vi "LinearRegression.vi"(8 "error in":errorcluster) -> (0 "error out":errorcluster, 3 "out":refnum<class "LinearRegression.lvclass">)   [LabVIEW 2020]
doc: "Ordinary least squares Linear Regression.\n\n LinearRegression fits a linear model with coefficients w = (w1, ..., wp)\n to minimize the residual sum of squares between the observed targets in\n the dataset, and the targets predicted by the linear approximation.\n\n Parameters\n ----------\n fit_intercept : bool, default=True\n Whether to calculate the intercept for this model. If set\n to False, no intercept will be used in calculations\n (i.e. data is expected to be centered).\n\n normalize : bool, default=False\n This parameter is ignored when ``fit_intercept`` is set to False.\n If True, the regressors X will be normalized before regression by\n subtracting the mean and dividing by the l2-norm.\n If you wish to standardize, please use\n :class:`~sklearn.preprocessing.StandardScaler` before calling ``fit``\n on an estimator with ``normalize=False``.\n\n copy_X : bool, default=True\n If True, X will be copied; else, it may be overwritten.\n\n n_jobs : int, default=None\n The number of jobs to use for the computation. This will only provide\n speedup for n_targets > 1 and sufficient large problems.\n ``None`` means 1 unless in a :obj:`joblib.parallel_backend` context.\n ``-1`` means using all processors. See :term:`Glossary <n_jobs>`\n for more details.\n\n positive : bool, default=False\n When set to ``True``, forces the coefficients to be positive. This\n option is only supported for dense arrays.\n\n .. versionadded:: 0.24\n\n Attributes\n ----------\n coef_ : array of shape (n_features, ) or (n_targets, n_features)\n Estimated coefficients for the linear regression problem.\n If multiple targets are passed during the fit (y 2D), this\n is a 2D array of shape (n_targets, n_features), while if only\n one target is passed, this is a 1D array of length n_features.\n\n rank_ : int\n Rank of matrix `X`. Only available when `X` is dense.\n\n singular_ : array of shape (min(X, y),)\n Singular values of `X`. Only available when `X` is dense.\n\n intercept_ : float or array of shape (n_targets,)\n Independent term in the linear model. Set to 0.0 if\n `fit_intercept = False`.\n\n See Also\n --------\n Ridge : Ridge regression addresses some of the\n problems of Ordinary Least Squares by imposing a penalty on the\n size of the coefficients with l2 regularization.\n Lasso : The Lasso is a linear model that estimates\n sparse coefficients with l1 regularization.\n ElasticNet : Elastic-Net is a linear regression\n model trained with both l1 and l2 -norm regularization of the\n coefficients.\n\n Notes\n -----\n From the implementation point of view, this is just plain Ordinary\n Least Squares (scipy.linalg.lstsq) or Non Negative Least Squares\n (scipy.optimize.nnls) wrapped as a predictor object.\n\n \nAvailable methods:\nGet Attributes\nGet Params\nSet Params"
uses:
  LinearRegression.lvclass
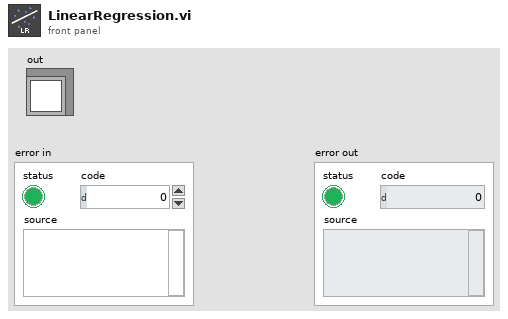
[diagram p1: front panel]
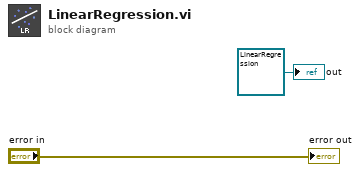
[diagram p0: block diagram]
diagram:
  "out" <- refnum<class "LinearRegression.lvclass"> refnum ("model")
  "error out" <- "error in"
